vi "Test_StartOfList_Wrap.vi"(8 "error in (no error)":errorcluster, 11 "TestCase in":refnum<class "TestStringList.lvclass">) -> (0 "error out":errorcluster, 3 "TestCase out":refnum<class "TestStringList.lvclass">)   [LabVIEW 2015, in "StringList.lvlib" / "TestStringList.lvclass"]
uses:
  TestStringList.lvclass
  <vilib>/addons/_JKI Toolkits/VI Tester/TestCase.llb/TestCase.lvclass
  StringList.lvclass
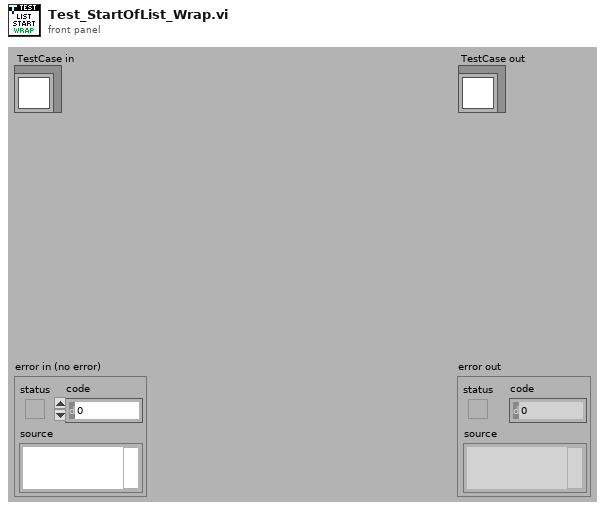
[diagram p1: front panel]
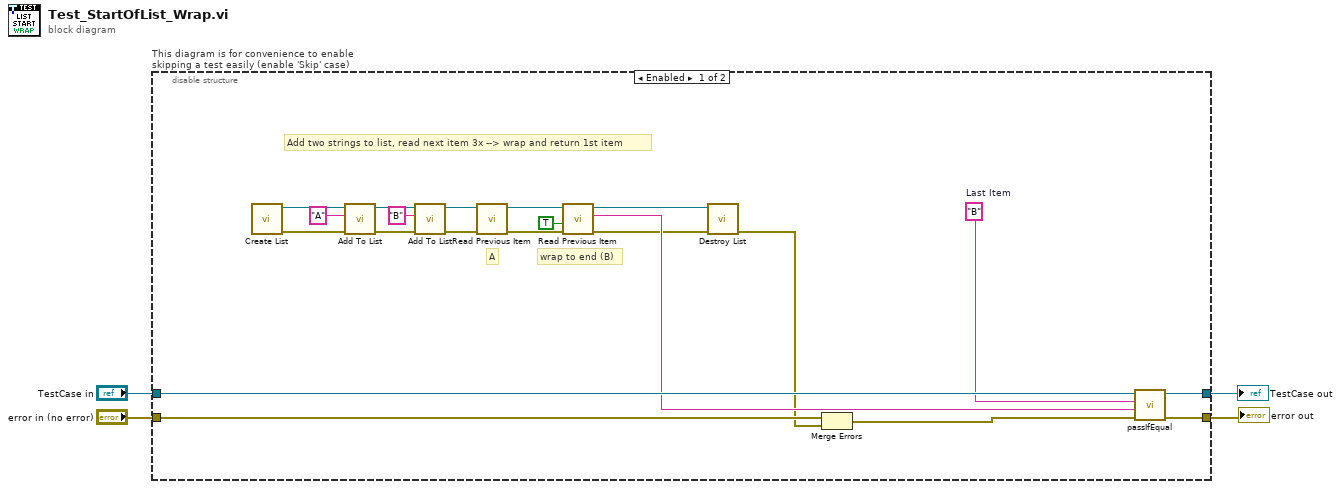
[diagram p0: block diagram]
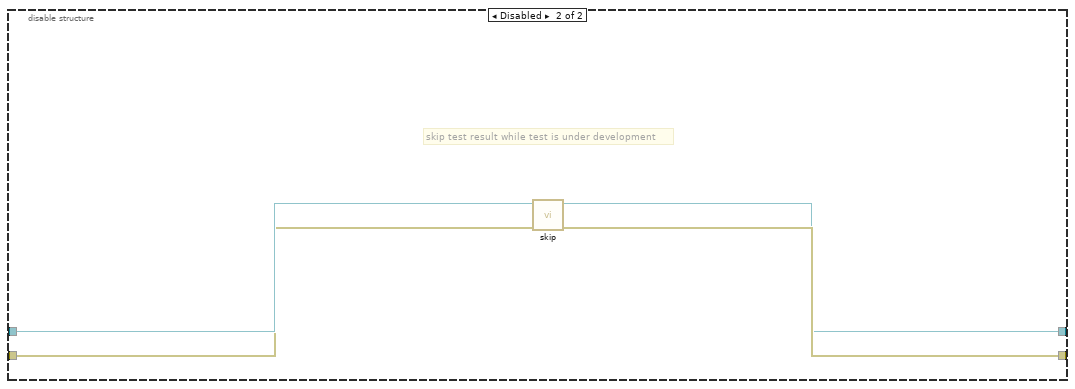
[diagram p2: hidden frame]
diagram:
  n1 = disable-structure "This diagram is for convenience to enable skipping a test easily (enable 'Skip' case)" shown="Enabled" {
    disable-tunnel: "TestCase in" -> [w25 w29]
    disable-tunnel: [w24 w27] -> w1
    disable-tunnel: [w23 w28] -> w3
    disable-tunnel: "error in (no error)" -> [w22 w26]
    frame Enabled {
      w21 = "B"  # Last Item
      # "wrap to end (B)"
      # "A"
      # "Add two strings to list, read next item 3x --> wrap and return 1st item"
      n2 = call "Create List.vi"() -> ("error out"=w11:errorcluster, "StringList Reference"=w17:refnum<data-value>)  [unwired: 10 in]
      n3 = call "Add To List.vi"("error in (no error)"=w11, "Item"="A", "StringList Reference"=w17) -> ("error out"=w10:errorcluster, "StringList Reference"=w20:refnum<data-value>)  [unwired: 7 in]
      n4 = call "Add To List.vi"("error in (no error)"=w10, "Item"="B", "StringList Reference"=w20) -> ("error out"=w9:errorcluster, "StringList Reference"=w16:refnum<data-value>)  [unwired: 7 in]
      n5 = call "Read Previous Item.vi"("error in (no error)"=w9, "StringList Reference"=w16) -> ("error out"=w8:errorcluster, "StringList Reference"=w18:refnum<data-value>)  [unwired: 6 in, 2 out]
      n6 = call "Read Previous Item.vi"("error in (no error)"=w8, "Wrap? (F)"=TRUE, "StringList Reference"=w18) -> ("error out"=w7:errorcluster, "Item"=w14:string, "StringList Reference"=w12:refnum<data-value>)  [unwired: 5 in, 1 out]
      n7 = call "Destroy List.vi"("error in (no error)"=w7, "StringList Reference"=w12) -> ("error out"=w5:errorcluster)  [unwired: 8 in, 1 out]
      n8 = Merge Errors(w22, w5) -> (w6:errorcluster)
      n9 = call-dynamic "passIfEqual.vi"("error in (no error)"=w6, "y"=w14, "x"=w21, "TestCase in"=w25) -> ("error out"=w23:errorcluster, "TestCase out"=w24:refnum<class "TestStringList.lvclass">)  [unwired: 6 in]
    }
    frame Disabled {
      # "skip test result while test is under development"
      n10 = call <vilib>:"skip.vi"("error in (no error)"=w26, "TestCase in"=w29) -> ("error out"=w28:errorcluster, "TestCase out"=w27:refnum<class "TestStringList.lvclass">)  [unwired: 8 in]
    }
  }
  "error out" <- w3
  "TestCase out" <- w1
